vi "Cleanup.vi"(8 "error in (no error)":errorcluster, 11 "Joystick in":refnum<class "Joystick.lvclass">) -> (0 "error out":errorcluster)   [LabVIEW 2020, in "Joystick.lvlib" / "Joystick.lvclass"]
doc: "Releases resources for an acquired Joystick instance. This should be called to ensure the joystick device can be used again if desired."
uses:
  Joystick.lvclass
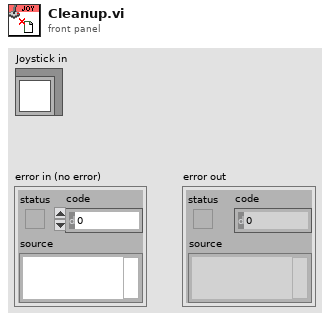
[diagram p1: front panel]
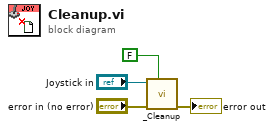
[diagram p0: block diagram]
diagram:
  n1 = call "_Cleanup.vi"("Skip Child?"=FALSE, "error in (no error)"="error in (no error)", "Joystick in"="Joystick in") -> ("error out"=→"error out":errorcluster)  [unwired: 8 in]
